vi "时间数据转换.vi"(7 "时间寄存器":u16[](array[numeric]) format="%04xH", 8 "error in (no error)":errorcluster caption="错误输入（无错误）", 11 "时间":timestamp) -> (0 "error out":errorcluster caption="错误输出", 3 "time stamp":timestamp)   [LabVIEW 2016, in "综合生物毒性.lvlib"]
uses:
  <vilib>/Utility/miscctls.llb/LVDateTimeRec.ctl
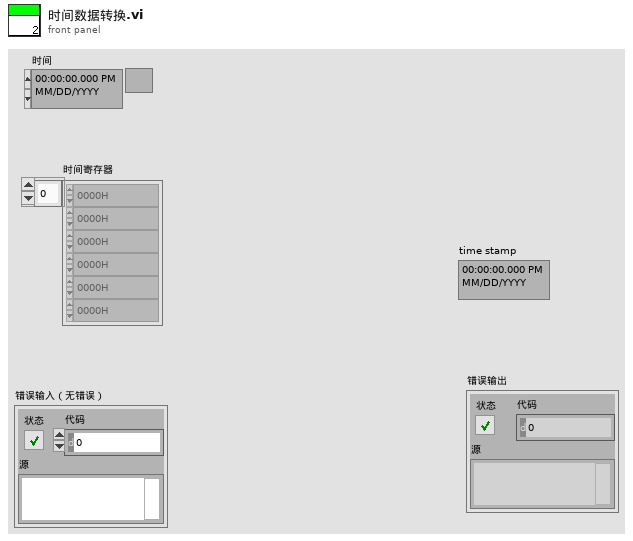
[diagram p1: front panel]
types:
  T1 = typedef "LVDateTimeRec.ctl" = cluster{"fractional second":dbl, "second":i32, "minute":i32, "hour":i32, "day of month":i32, "month":i32, "year":i32, "day of week":i32, "day of year":i32, "DST":i32}
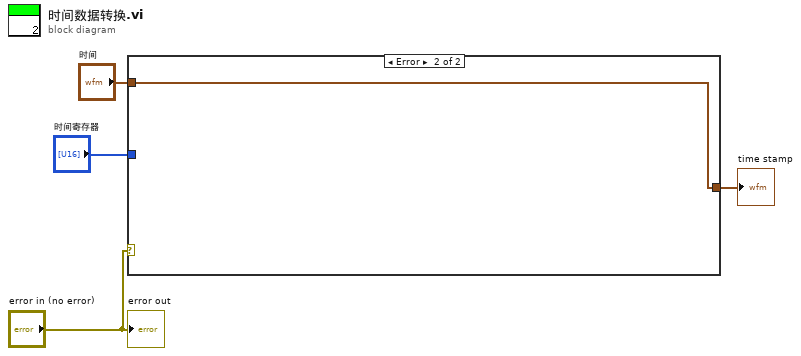
[diagram p0: block diagram]
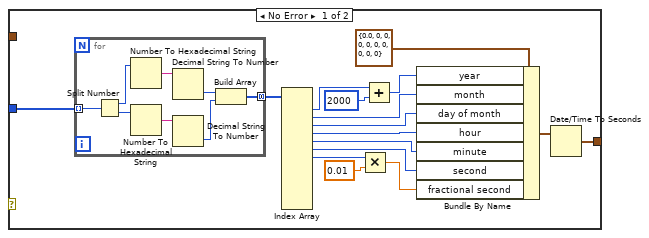
[diagram p2: hidden frame]
diagram:
  n1 = case shown="Error" "error in (no error)" {
    tunnel: "时间寄存器" -> [w20 _]
    tunnel: [w8 w29] -> w3
    tunnel: "时间" -> [_ w29]
    frame No Error {
      n2 = for {
        tunnel: w20 -> [w28] mode=indexing
        tunnel: [w25] -> w19 mode=concatenating
        n3 = Split Number(x=w28) -> (hi(x)=w24:u8, lo(x)=w22:u8)
        n4 = Number To Hexadecimal String(2:w24) -> (0:w23:string)  [unwired: 1 in]
        n5 = Number To Hexadecimal String(2:w22) -> (0:w21:string)  [unwired: 1 in]
        n6 = Decimal String To Number(string=w23) -> (number=w27:i32)  [unwired: 2 in, 1 out]
        n7 = Decimal String To Number(string=w21) -> (number=w26:i32)  [unwired: 2 in, 1 out]
        n8 = Build Array(w27, w26) -> (w25:i32[])
      }
      n9 = Index Array(array=w19) -> (element #1=w7:i32, element #2=w17:i32, element #3=w16:i32, element #4=w15:i32, element #5=w14:i32, element #6=w13:i32, element #7=w12:i32)  [unwired: 13 in, 6 out]
      n10 = Multiply(x=w12, y=0.01) -> (x*y=w10:dbl)
      n11 = Add(x=w7, y=2000) -> (x+y=w5:i32)
      n12 = Bundle By Name(cluster=T1 {"fractional second"=0.0, "second"=0, "minute"=0, "hour"=0, "day of month"=0, "month"=0, "year"=0, "day of week"=0, "day of year"=0, "DST"=0} ("日期时间记录"), "year"=w5, "month"=w17, "day of month"=w16, "hour"=w15, "minute"=w14, "second"=w13, "fractional second"=w10) -> (w9:T1)
      n13 = Date/Time To Seconds(2:w9) -> (0:w8:timestamp)  [unwired: 1 in]
    }
    frame Error {
    }
  }
  "time stamp" <- w3
  "error out" <- "error in (no error)"
